vi "GlobalLaserInterface.vi"() -> ()   [LabVIEW 2009]
panel:
  in  "InterfaceLaserInitalised":refnum<visa-resource-name>
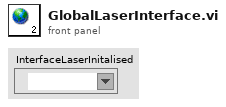
[diagram p1: front panel]
diagram:
